vi "反馈节点 2.vi"() -> ()   [LabVIEW 2023]
panel:
  out "Array 2":i32[][](array[numeric])
  out "Array":i32[](array[numeric])
  out "x+y 2":i32
  out "x+y":i32
  # "反馈节点 2"
  # "在多层嵌套循环中，反馈节点会被包含它的每一层循环结构调用。\n它相当于在包含它的每一层循环结构上都建立了一对移位寄存器，然后把它们串联起来。"
  # "例子一"
  # "例子2"
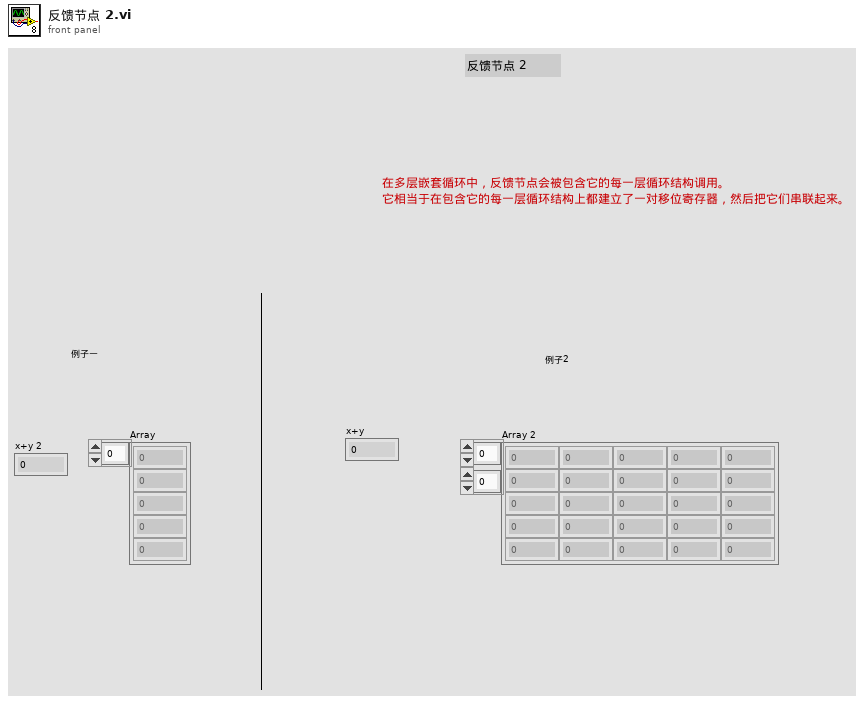
[diagram p1: front panel]
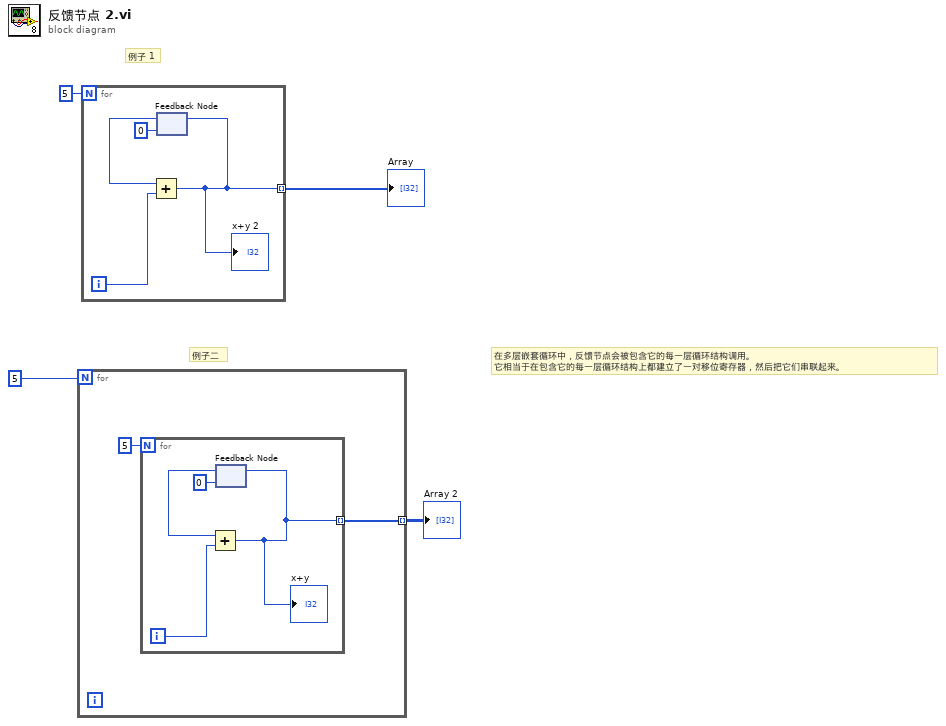
[diagram p0: block diagram]
diagram:
  # "在多层嵌套循环中，反馈节点会被包含它的每一层循环结构调用。\n它相当于在包含它的每一层循环结构上都建立了一对移位寄存器，然后把它们串联起来。"
  # "例子二"
  # "例子 1"
  n1 = for {
    N: 5 -> [_]
    tunnel: [w5] -> w1 mode=indexing
    n2 = for {
      N: 5 -> [_]
      tunnel: [w7] -> w5 mode=indexing
      i -> [w10]
      n3 = feedback #1(0) -> (w9:i32)
      n4 = Add(x=w9, y=w10) -> (x+y=w7:i32)
      "x+y" <- w7
      n5 = feedback-in #1(w7) -> ()
    }
  }
  "Array 2" <- w1
  n6 = for {
    N: 5 -> [_]
    tunnel: [w11] -> w2 mode=indexing
    i -> [w14]
    n7 = feedback #2(0) -> (w13:i32)
    n8 = Add(x=w13, y=w14) -> (x+y=w11:i32)
    "x+y 2" <- w11
    n9 = feedback-in #2(w11) -> ()
  }
  "Array" <- w2
